vi "Logitech F310.vi"(6 "error in (no error)":errorcluster, 7 "Deadzone Scale Cluster":cluster{"Scale":dbl, "Deadzone":dbl}, 8 "refnum name":string) -> (0 "Buttons":T2, 1 "D-Pad Buttons":T1, 2 "D-Pad":cluster{"X":dbl, "Y":dbl}, 3 "Right Stick":cluster{"X":dbl, "Y":dbl}, 4 "error out":errorcluster, 5 "Left Stick":cluster{"X":dbl, "Y":dbl})   [LabVIEW 2014]
uses:
  <vilib>/Rock Robotics/WPI/Joystick/WPI_JoystickGetSetRefNum.vi
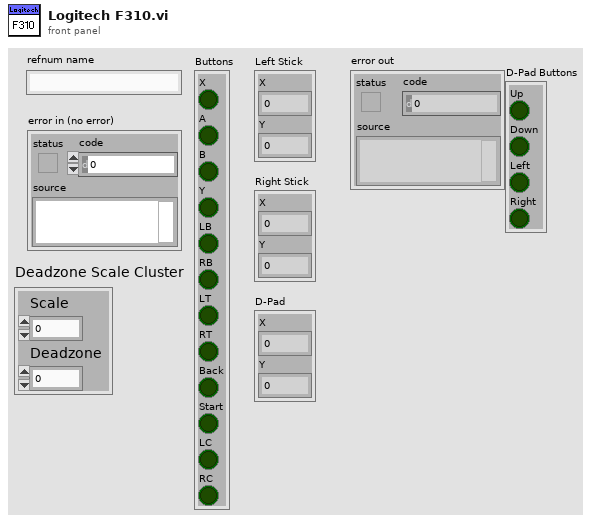
[diagram p1: front panel]
types:
  T1 = cluster{"Up":bool, "Down":bool, "Left":bool, "Right":bool}
  T2 = cluster{"X":bool, "A":bool, "B":bool, "Y":bool, "LB":bool, "RB":bool, "LT":bool, "RT":bool, "Back":bool, "Start":bool, "LC":bool, "RC":bool}
  T3 = typedef "WPI_JoystickDevRef.ctl" = cluster{"Device":T4}
  T4 = typedef "WPI_JoystickDeviceEnum.ctl" = enum16{"USB 0", "USB 1", "USB 2", "USB 3", "USB 4", "USB 5"}
  T5 = cluster{"Button 1":bool, "Button 2":bool, "Button 3":bool, "Button 4":bool, "Button 5":bool, "Button 6":bool, "Button 7":bool, "Button 8":bool, "Button 9":bool, "Button 10":bool, "Button 11":bool, "Button 12":bool}
  T6 = cluster{"axis 1 (x)":dbl, "axis 2 (y)":dbl, "axis 3 (throttle)":dbl, "axis 4":dbl, "axis 5":dbl, "axis 6":dbl}
  T7 = cluster{"[0]":dbl, "[1]":dbl, "[2]":dbl, "[3]":dbl, "[4]":dbl, "[5]":dbl}
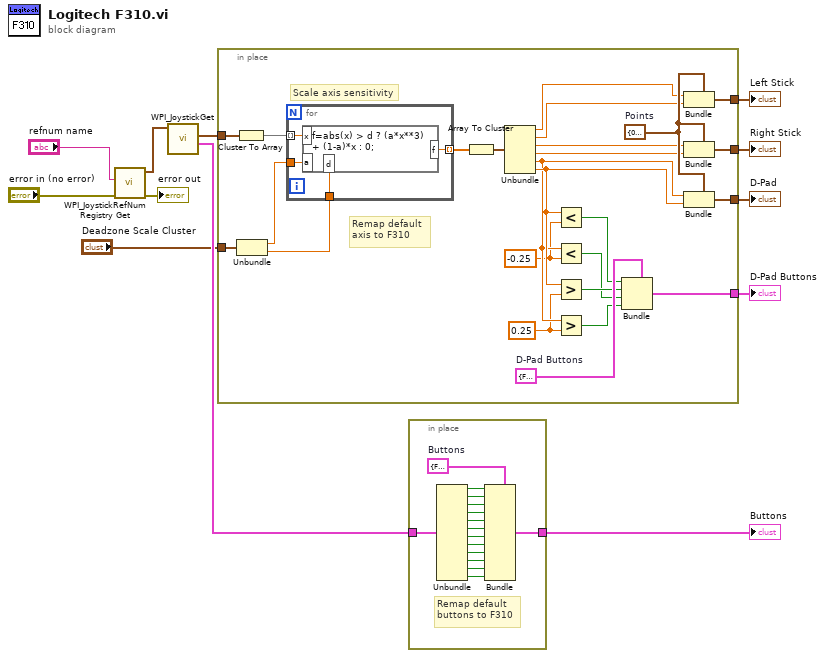
[diagram p0: block diagram]
diagram:
  n1 = call <vilib>:"WPI_JoystickRefNum Registry Get.vi"("error in (no error)"="error in (no error)", "refnum name"="refnum name") -> ("error out"=→"error out":errorcluster, "JoystickDevRef"=w12:T3)  [unwired: 8 in]
  n2 = call <vilib>:"WPI_JoystickGet.vi"("JoystickDevRef"=w12) -> ("Buttons"=w10:T5, "Axes"=w11:T6)  [unwired: 4 in, 1 out]
  n3 = in-place {
    in-place-border: w11 -> [w19]
    in-place-border: [w37] -> w6
    in-place-border: [w36] -> w5
    in-place-border: [w34] -> w4
    in-place-border: [w28] -> w2
    in-place-border: "Deadzone Scale Cluster" -> [w15]
    w29 = -0.25 ("y")
    w30 = 0.25 ("y")
    w33 = T1 {"Up"=FALSE, "Down"=FALSE, "Left"=FALSE, "Right"=FALSE}  # D-Pad Buttons
    w35 = cluster{"X":dbl, "Y":dbl} {"X"=0.0, "Y"=0.0}  # Points
    # "Scale axis sensitivity"
    # "Remap default\naxis to F310"
    n4 = Cluster To Array(cluster=w19) -> (array=w17:dbl[])
    n5 = Unbundle(w15) -> ("Scale"=w14:dbl, "Deadzone"=w13:dbl)
    n6 = for {
      tunnel: w17 -> [w41] mode=indexing
      tunnel: [w40] -> w16 mode=indexing
      tunnel: w14 -> [w39]
      tunnel: w13 -> [w38]
      n7 = formula code="f=abs(x) > d ? (a*x**3) + (1-a)*x : 0;"("x"=w41, "a"=w39, "d"=w38) -> ("f"=w40:dbl)
    }
    n8 = Array To Cluster(array=w16) -> (cluster=w18:T7)
    n9 = Unbundle(w18) -> ("[0]"=w23:dbl, "[1]"=w22:dbl, "[2]"=w21:dbl, "[3]"=w20:dbl, "[4]"=w31:dbl, "[5]"=w32:dbl)
    n10 = Less?(x=w32, y=w29) -> (x < y?=w26:bool)
    n11 = Less?(x=w31, y=w29) -> (x < y?=w24:bool)
    n12 = Greater?(x=w32, y=w30) -> (0:w27:bool)
    n13 = Greater?(x=w31, y=w30) -> (0:w25:bool)
    n14 = Bundle(cluster=w33, "Up"=w26, "Down"=w27, "Left"=w24, "Right"=w25) -> (w28:T1)
    n15 = Bundle(cluster=w35, "X"=w23, "Y"=w22) -> (w37:cluster{"X":dbl, "Y":dbl})
    n16 = Bundle(cluster=w35, "X"=w21, "Y"=w20) -> (w36:cluster{"X":dbl, "Y":dbl})
    n17 = Bundle(cluster=w35, "X"=w31, "Y"=w32) -> (w34:cluster{"X":dbl, "Y":dbl})
  }
  "Left Stick" <- w6
  "Right Stick" <- w5
  "D-Pad" <- w4
  "D-Pad Buttons" <- w2
  n18 = in-place {
    in-place-border: w10 -> [w56]
    in-place-border: [w42] -> w3
    w55 = T2 {"X"=FALSE, "A"=FALSE, "B"=FALSE, "Y"=FALSE, "LB"=FALSE, "RB"=FALSE, "LT"=FALSE, "RT"=FALSE, "Back"=FALSE, "Start"=FALSE, "LC"=FALSE, "RC"=FALSE}  # Buttons
    # "Remap default\nbuttons to F310"
    n19 = Unbundle(w56) -> ("Button 1"=w54:bool, "Button 2"=w53:bool, "Button 3"=w52:bool, "Button 4"=w51:bool, "Button 5"=w50:bool, "Button 6"=w49:bool, "Button 7"=w48:bool, "Button 8"=w47:bool, "Button 9"=w46:bool, "Button 10"=w45:bool, "Button 11"=w44:bool, "Button 12"=w43:bool)
    n20 = Bundle(cluster=w55, "X"=w54, "A"=w53, "B"=w52, "Y"=w51, "LB"=w50, "RB"=w49, "LT"=w48, "RT"=w47, "Back"=w46, "Start"=w45, "LC"=w44, "RC"=w43) -> (w42:T2)
  }
  "Buttons" <- w3
